vi "DSF.Engine.Plugin.Get Timing.vi"(11 "Plugin in":refnum<class "DSF.Engine.Plugin.lvclass">) -> (2 "Timing":refnum<class "DSF.Shared.Timing.lvclass">, 3 "Plugin out":refnum<class "DSF.Engine.Plugin.lvclass">)   [LabVIEW 2017, in "DSF.Engine.lvlib" / "DSF.Engine.Plugin.lvclass"]
uses:
  DSF.Engine.Plugin.lvclass
  Shared/Classes/Timing/DSF.Shared.Timing.lvclass
  DSF.Engine.Plugin.lvclass/DSF.Engine.Plugin.ctl
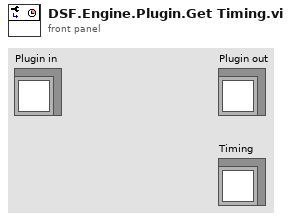
[diagram p1: front panel]
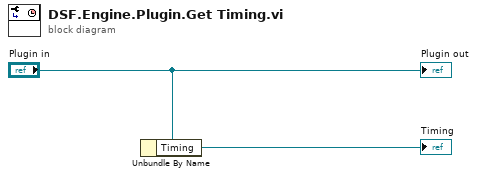
[diagram p0: block diagram]
diagram:
  n1 = Unbundle By Name("Plugin in") -> ("Timing"=→"Timing":refnum<class "DSF.Shared.Timing.lvclass">)
  "Plugin out" <- "Plugin in"
